vi "Connection Test App.vi"   [LabVIEW 2011]
uses:
  LVH-LINX.lvlib
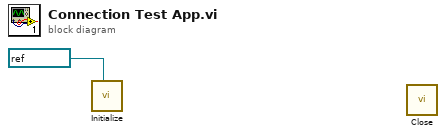
[diagram p0: block diagram]
diagram:
  n1 = call "Initialize.vi"("Serial Port"=refnum<visa-resource-name> "COM7") -> ()  [unwired: 9 in, 2 out]
  n2 = call "Close.vi"() -> ()  [unwired: 12 in]
